vi "Block_No_Av.vi"(2 "Raw data file":path, 3 "Results file":path) -> ()   [LabVIEW 2011]
uses:
  Controls/Save_Data.ctl
  Controls/Setup.ctl
  Controls/Post_Process.ctl
  Block_Control_global.vi
  Globals/Meas_global.vi
panel:
  in  "Desired Averaging Time (mins)":dbl=5.0
  out "Current Row Number":i32
  out "No of Rows":i32
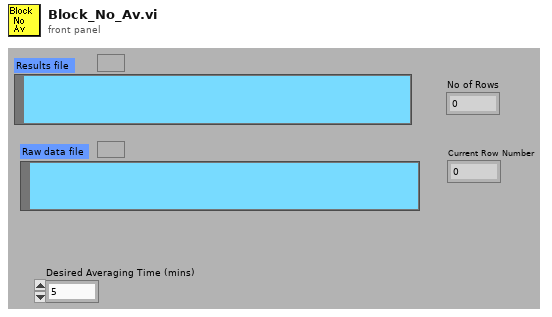
[diagram p1: front panel]
types:
  T1 = typedef "Save_Data.ctl" = enum16{"Save No Data", "Save Data"}
  T2 = typedef "Setup.ctl" = enum16{"Run Program", "Show Setup", "Save Current Setup", "Setup Front Panel"}
  T3 = typedef "Post_Process.ctl" = enum16{"Take New Data", "Post Process Raw Data File"}
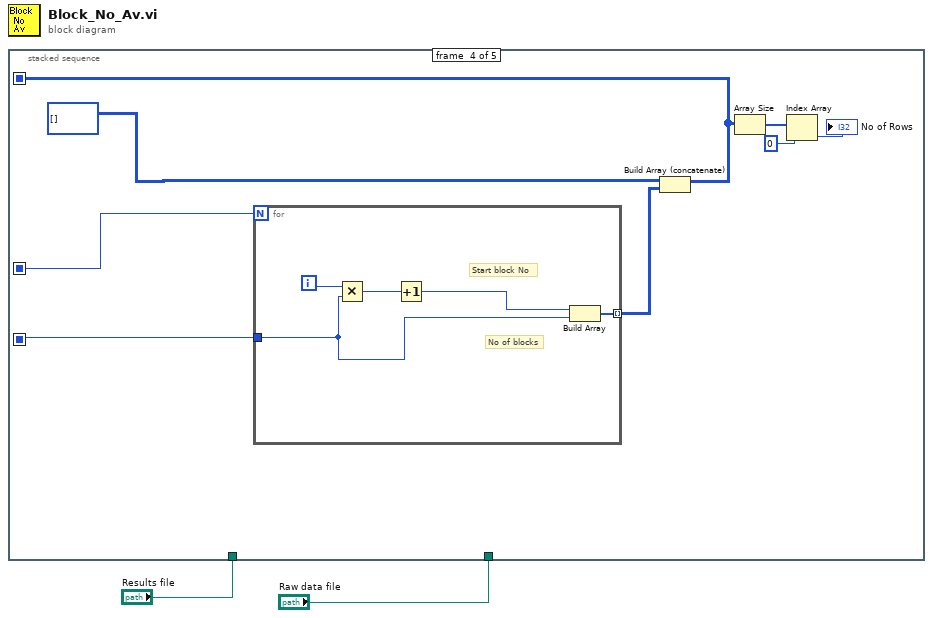
[diagram p0: block diagram]
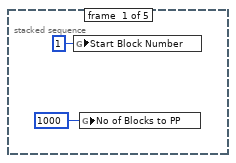
[diagram p2: hidden frame]
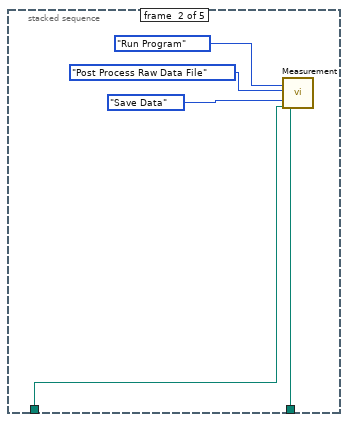
[diagram p3: hidden frame]
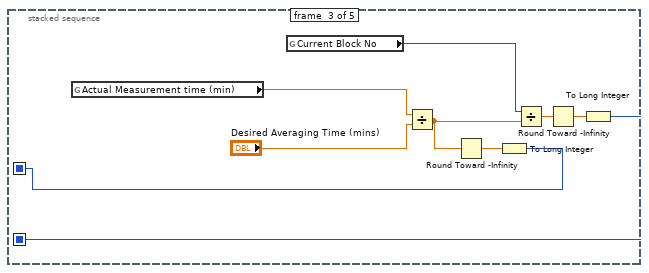
[diagram p4: hidden frame]
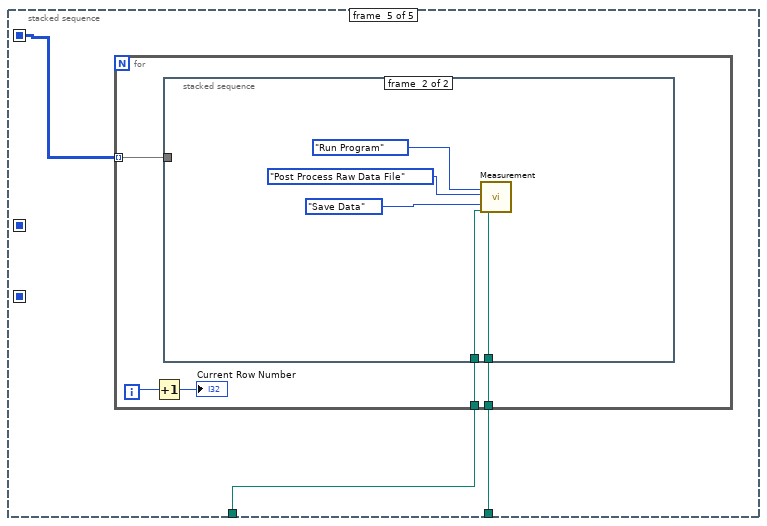
[diagram p5: hidden frame]
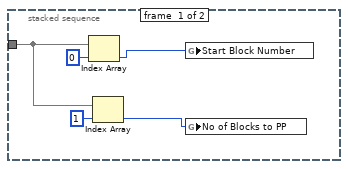
[diagram p6: hidden frame]
diagram:
  n1 = stacked-sequence {
    seq-local: [_ _ _ w22 _] -> [_ _ _ _ w32]
    seq-local: [_ _ w10 _ _] -> [_ _ _ w19 _]
    seq-local: [_ _ w11 _ _] -> [_ _ _ w20 _]
    tunnel: "Raw data file" -> [_ w7 _ _ w34]
    tunnel: "Results file" -> [_ w6 _ _ w33]
    frame #0 {
      n2 = global write "Block_Control_global.vi" "Start Block Number"(1 ("Start Block Number")) -> ()
      n3 = global write "Block_Control_global.vi" "No of Blocks to PP"(1000 ("Start Block Number")) -> ()
    }
    frame #1 {
      n4 = call "Measurement.vi"("setup"=Setup."Run Program", "Post Process"=Post_Process."Post Process Raw Data File", "File"=Save_Data."Save Data", "Results file"=w6, "Raw data file"=w7) -> ()  [unwired: 2 in, 13 out]
    }
    frame #2 {
      n5 = global read "Meas_global.vi" "Actual Measurement time (min)"() -> (w18:dbl)
      n6 = global read "Meas_global.vi" "Current Block No"() -> (w16:i32)
      n7 = Divide(x=w18, y="Desired Averaging Time (mins)") -> (x/y=w15:dbl)
      n8 = Round Toward -Infinity(1:w15) -> (0:w14:dbl)
      n9 = To Long Integer(number=w14) -> (32bit integer=w10:i32)
      n10 = Divide(x=w16, y=w15) -> (x/y=w13:dbl)
      n11 = Round Toward -Infinity(1:w13) -> (0:w12:dbl)
      n12 = To Long Integer(number=w12) -> (32bit integer=w11:i32)
    }
    frame #3 {
      n13 = for {
        N: w19 -> [_]
        tunnel: [w31] -> w21 mode=indexing
        tunnel: w20 -> [w27]
        i -> [w29]
        # "Start block No"
        # "No of blocks"
        n14 = Multiply(x=w29, y=w27) -> (x*y=w30:i32)
        n15 = Increment(x=w30) -> (x+1=w28:i32)
        n16 = Build Array(w28, w27) -> (w31:i32[])
      }
      n17 = Build Array (concatenate)(i32[][] [], w21) -> (w22:i32[][])
      n18 = Array Size(array=w22) -> (size(s)=w25:i32[])
      n19 = Index Array(array=w25, index=0) -> (element=→"No of Rows":i32)
    }
    frame #4 {
      n20 = for {
        tunnel: w34 -> [w39]
        tunnel: w33 -> [w38]
        tunnel: w32 -> [w37] mode=indexing
        i -> [w36]
        n21 = Increment(x=w36) -> (x+1=→"Current Row Number":i32)
        n22 = stacked-sequence {
          tunnel: w39 -> [_ w47]
          tunnel: w38 -> [_ w46]
          tunnel: w37 -> [w42 _]
          frame #0 {
            n23 = Index Array(array=w42, index=0) -> (element=w40:i32)
            n24 = Index Array(array=w42, index=1) -> (element=w41:i32)
            n25 = global write "Block_Control_global.vi" "Start Block Number"(w40) -> ()
            n26 = global write "Block_Control_global.vi" "No of Blocks to PP"(w41) -> ()
          }
          frame #1 {
            n27 = call "Measurement.vi"("setup"=Setup."Run Program", "Post Process"=Post_Process."Post Process Raw Data File", "File"=Save_Data."Save Data", "Results file"=w46, "Raw data file"=w47) -> ()  [unwired: 2 in, 13 out]
          }
        }
      }
    }
  }
